vi "Generate Test Server.vi"(1 "Connection Configuration":T2, 3 "error in (no error)":errorcluster) -> (7 "OPC UA server refnum out":refnum<k21>, 8 "server endpoint URL":string, 10 "error out":errorcluster)   [LabVIEW 2013, in "OPC UA Client Tests.lvlib"]
doc: "Generate OPC UA Server for Tests\n\nThis is for testing purposes, is not robust and should not be used as part of the module itself."
uses:
  OPC UA Client Tests.lvlib
  <vilib>/OPCUA/server/subVI/supported security policies.ctl
  <vilib>/opcua/NI OPC UA Server.lvlib
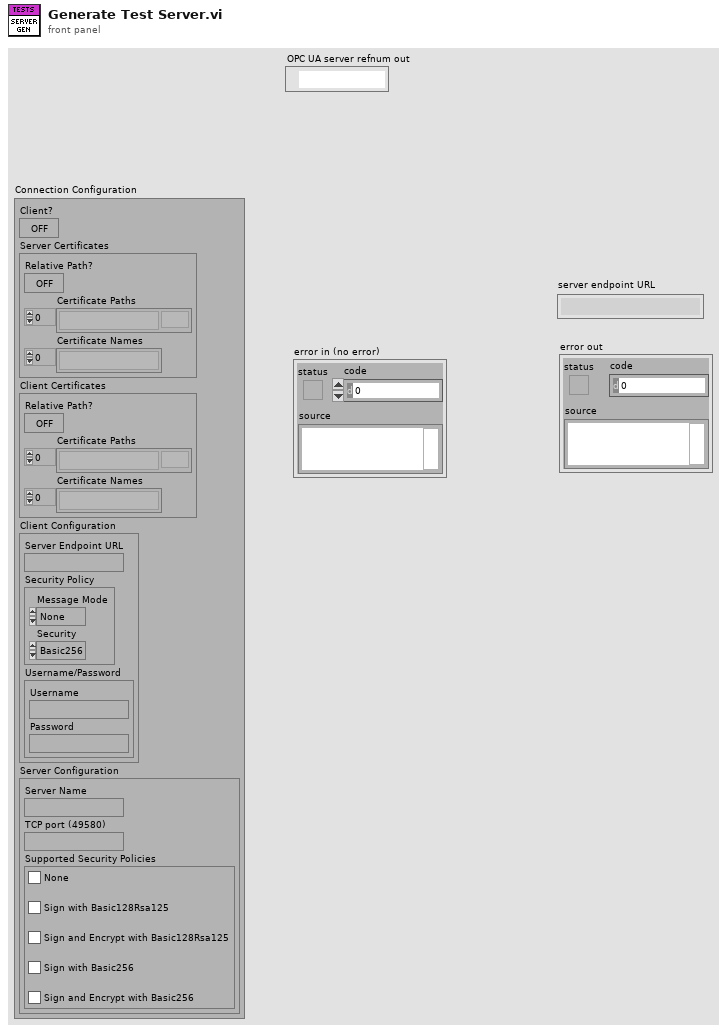
[diagram p1: front panel]
types:
  T1 = typedef "supported security policies.ctl" = cluster{"None":bool, "Sign with Basic128Rsa125":bool, "Sign and Encrypt with Basic128Rsa125":bool, "Sign with Basic256":bool, "Sign and Encrypt with Basic256":bool}
  T2 = cluster{"Client?":bool, "Server Certificates":cluster{"Relative Path?":bool, "Certificate Paths":path[], "Certificate Names":string[]}, "Client Certificates":cluster{"Relative Path?":bool, "Certificate Paths":path[], "Certificate Names":string[]}, "Client Configuration":cluster{"Server Endpoint URL":string, "Security Policy":cluster{"Message Mode":enum16{"None", "Sign", "Sign and Encrypt"}, "Security":enum16{"Basic256", "Basic128Rsa15"}}, "Username/Password":cluster{"Username":string, "Password":string}}, "Server Configuration":cluster{"Server Name":string, "TCP port (49580)":string, "Supported Security Policies":T1}}
  T3 = cluster{"Relative Path?":bool, "Certificate Paths":path[], "Certificate Names":string[]}
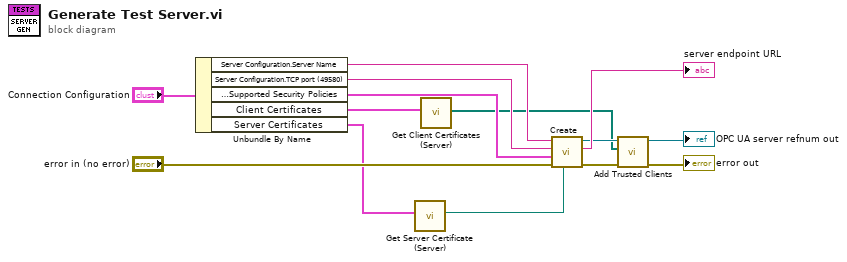
[diagram p0: block diagram]
diagram:
  n1 = Unbundle By Name("Connection Configuration") -> ("Server Configuration.Server Name"=w8:string, "Server Configuration.TCP port (49580)"=w7:string, "Server Configuration.Supported Security Policies"=w6:T1, "Client Certificates"=w5:T3, "Server Certificates"=w3:T3)
  n2 = call "Get Server Certificate (Server).vi"("Server Certificates"=w3) -> ("server certificate file"=w2:path)  [unwired: 10 in]
  n3 = call "Get Client Certificates (Server).vi"("Client Certificates"=w5) -> ("trusted client certificates"=w4:path[])  [unwired: 10 in]
  n4 = call <vilib>:"Create.vi"("server certificate file"=w2, "error in (no error)"="error in (no error)", "supported security policies (None)"=w6, "TCP port (49580)"=w7, "OPC UA server name"=w8) -> ("error out"=w11:errorcluster, "server endpoint URL"=→"server endpoint URL":string, "OPC UA server refnum out"=w12:refnum<k21>)  [unwired: 4 in]
  n5 = call <vilib>:"Add Trusted Clients.vi"("error in (no error)"=w11, "trusted client certificates"=w4, "OPC UA server refnum in"=w12) -> ("error out"=→"error out":errorcluster, "OPC UA server refnum out"=→"OPC UA server refnum out":refnum<k21>)  [unwired: 7 in]
